vi "Write ini file path.vi"(8 "error in (no error)":errorcluster, 10 "ini file path":path, 11 "Standard in":refnum<class "Standard.lvclass">) -> (0 "error out":errorcluster, 3 "Standard out":refnum<class "Standard.lvclass">)   [LabVIEW 2018, in "Standard.lvclass"]
uses:
  Standard.lvclass
  Standard.lvclass/Standard.ctl
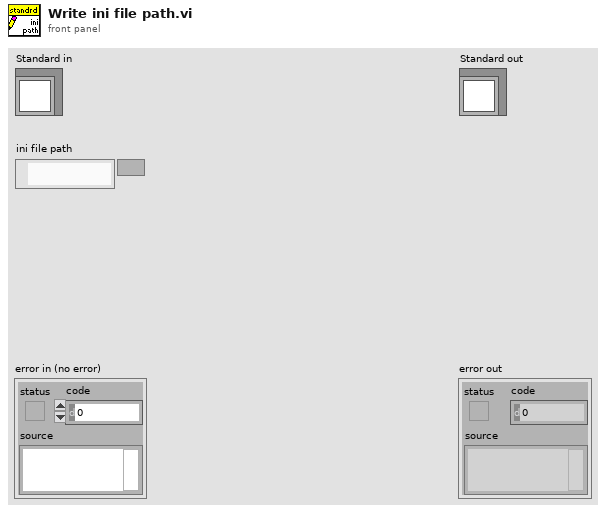
[diagram p1: front panel]
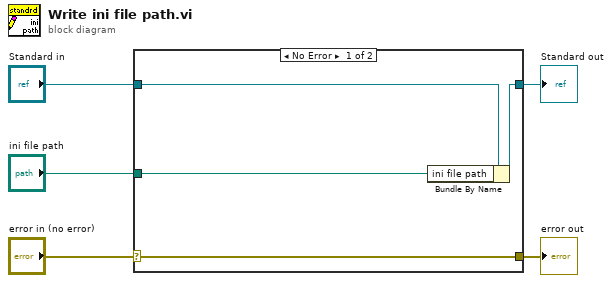
[diagram p0: block diagram]
diagram:
  n1 = case shown="No Error" "error in (no error)" {
    selector: "error in (no error)" -> [w9 w10]
    tunnel: [w9 w10] -> w4
    tunnel: [w7 w11] -> w2
    tunnel: "Standard in" -> [w8 w11]
    tunnel: "ini file path" -> [w6 _]
    frame No Error {
      n2 = Bundle By Name(cluster=w8, "ini file path"=w6) -> (w7:refnum<class "Standard.lvclass">)
    }
    frame Error {
    }
  }
  "error out" <- w4
  "Standard out" <- w2
